vi "main.vi"(9 "handler properties":T1={"max url size"=8000, "max header"=8000, "timeout ms"=5000, "max data size"=104857600}, 10 "connection handler pool size":i32=10, 11 "port":u16=80) -> (0 "error out":errorcluster)   [LabVIEW 2013]
uses:
  HTTP server/http server properties.ctl
  tests/ws console/Websocket console plugin.lvclass
  tests/test responder/test responder.lvclass
  HTTP responder/http responder.lvclass
  websocket/websocket upgrade handler.lvclass
  HTTP server/Basic HTTP server.lvclass
panel:
  in  "stop":bool
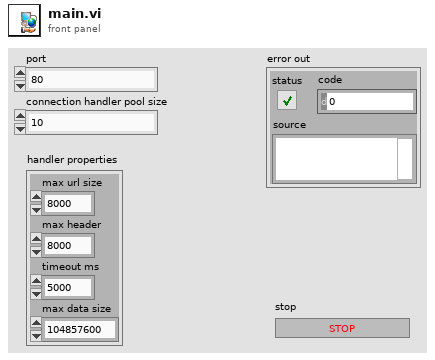
[diagram p1: front panel]
types:
  T1 = typedef "Basic HTTP server.lvclass/http server properties.ctl" = cluster{"max url size":i32, "max header":i32, "timeout ms":i32, "max data size":i32}
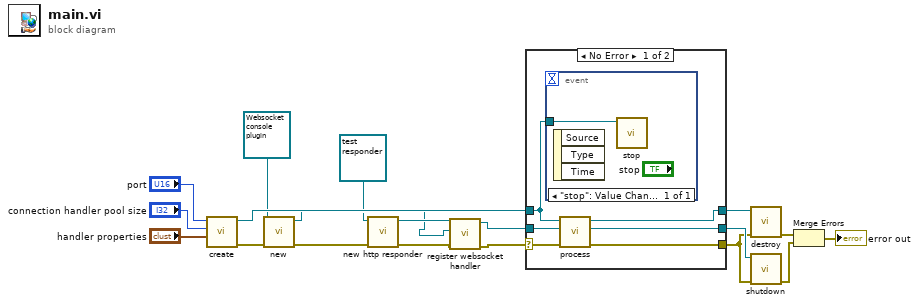
[diagram p0: block diagram]
diagram:
  n1 = call "create.vi"("handler properties"="handler properties", "connection handler pool size"="connection handler pool size", "port"="port") -> ("error out"=w10:errorcluster, "Basic HTTP server out"=w16:refnum<class "Basic HTTP server.lvclass">)  [unwired: 7 in]
  n2 = call-dynamic "new.vi"("error in"=w10, "Websocket console plugin in"=refnum<class "Websocket console plugin.lvclass"> refnum ("Websocket console plugin")) -> ("error out"=w6:errorcluster, "Websocket console plugin out"=w3:refnum<class "Websocket console plugin.lvclass">)  [unwired: 8 in]
  n3 = call-dynamic "new http responder.vi"("error in"=w6, "http responder in"=refnum<class "test responder.lvclass"> refnum ("test responder.lvclass")) -> ("error out"=w8:errorcluster, "http responder out"=w4:refnum<class "test responder.lvclass">)  [unwired: 8 in]
  n4 = call "register websocket handler.vi"("error in"=w8, "websocket user plugin"=w3, "http responder in"=w4) -> ("error out"=w7:errorcluster, "http responder out"=w5:refnum<class "test responder.lvclass">)  [unwired: 7 in]
  n5 = case shown="No Error" w7 {
    selector: w7 -> [w22 w28]
    tunnel: w16 -> [w25 w29]
    tunnel: [w24 w29] -> w15
    tunnel: [w23 w27] -> w14
    tunnel: w5 -> [w21 w27]
    tunnel: [w20 w28] -> w9
    frame No Error {
      n6 = event shown="[0] \"stop\": Value Change" {
        selector: _ -> [_]
        dyn-events: _ -> [_]
        timeout: _ -> [_]
        tunnel: w25 -> [w26]
        event "stop": Value Change {
          n7 = event-data() -> ()  [unwired: 1 in, 3 out]
          n8 = call "stop.vi"("Basic HTTP server in"=w26) -> ()  [unwired: 10 in, 1 out]
        }
      }
      n9 = call "process.vi"("error in"=w22, "responder in"=w21, "Basic HTTP server in"=w25) -> ("error out"=w20:errorcluster, "responder out"=w23:refnum<class "test responder.lvclass">, "Basic HTTP server out"=w24:refnum<class "Basic HTTP server.lvclass">)  [unwired: 6 in]
    }
    frame Error {
    }
  }
  n10 = call "destroy.vi"("error in"=w9, "Basic HTTP server in"=w15) -> ("error out"=w11:errorcluster)  [unwired: 9 in]
  n11 = call "shutdown.vi"("error in"=w9, "http responder in"=w14) -> ("error out"=w12:errorcluster)  [unwired: 9 in]
  n12 = Merge Errors(w11, w12) -> (→"error out":errorcluster)
